vi "FillLocalArray.vi"(4 "Sequence Context":refnum<k7>) -> (0 "error out":errorcluster)   [LabVIEW 2011]
doc: "Generates an array of data and writes it to a TestStand Local Variable using the TestStand Utility VIs."
uses:
  <vilib>/addons/TestStand/_TSUtility.llb/TestStand - Get Property Value (Numeric Array).vi
  <vilib>/addons/TestStand/_TSUtility.llb/TestStand - Set Property Value (Numeric Array).vi
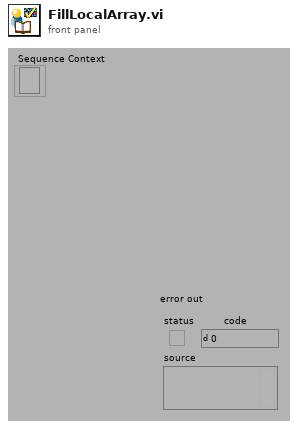
[diagram p1: front panel]
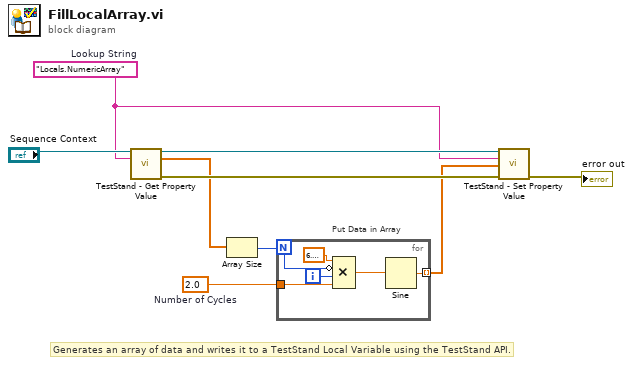
[diagram p0: block diagram]
diagram:
  w2 = 2.0  # Number of Cycles
  w4 = "Locals.NumericArray"  # Lookup String
  # "Generates an array of data and writes it to a TestStand Local Variable using the TestStand API."
  # "Put Data in Array"
  n1 = call-poly <vilib>:"TestStand - Get Property Value.vi"("Sequence Context In"="Sequence Context", "Lookup String"=w4) -> ("Sequence Context Out"=w6:refnum<k7>, "Value"=w5:dbl[], "error out"=w7:errorcluster)  [unwired: 1 in, 10 out]
  n2 = Array Size(array=w5) -> (size(s)=w3:i32)
  n3 = for {
    N: w3 -> [w13]
    tunnel: [w15] -> w1 mode=indexing
    tunnel: w2 -> [w11]
    i -> [w12]
    n4 = Compound Arithmetic op=MULTIPLY(6.283185307179586, invert w13, w12, w11) -> (w10:dbl)
    n5 = Sine(x=w10) -> (sin(x)=w15:dbl)
  }
  n6 = call-poly <vilib>:"TestStand - Set Property Value.vi"("Sequence Context In"=w6, "Lookup String"=w4, "New Value"=w1, "error in (no error)"=w7) -> ("error out"=→"error out":errorcluster)  [unwired: 1 in, 10 out]
